vi "Drive_Speed_Set(EEPRM).vi"(1 "Set Speed":i32, 2 "Drive Speed Number":u16(ring) items=["Drive Speed 1", "Drive Speed 2", "Drive Speed 3", "Drive Speed 4"], 3 "Axis":u16(ring) items=["X", "Y"], 4 "baud rate (9600)":u32=115200 caption="보 전송속도(9600)", 5 "Port":refnum<visa-resource-name>="COM4" caption="VISA 리소스 이름") -> (0 "Read Speed":u32)   [LabVIEW 2016]
uses:
  <vilib>/Instr/_visa.llb/VISA Configure Serial Port (Instr).vi
  <vilib>/Instr/_visa.llb/VISA Flush IO Buffer Mask.ctl
panel:
  out "Read Buffer":string
  out "VISA 리소스 이름 출력":refnum<visa-resource-name>
  out "에러 출력":errorcluster
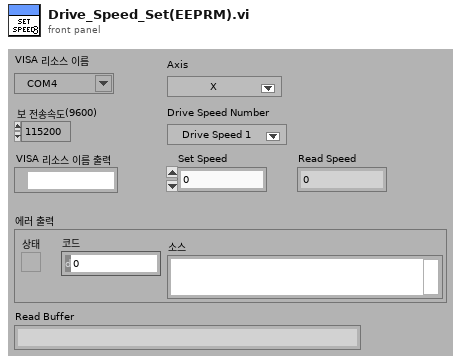
[diagram p1: front panel]
types:
  T1 = typedef "VISA Flush IO Buffer Mask.ctl" = u16
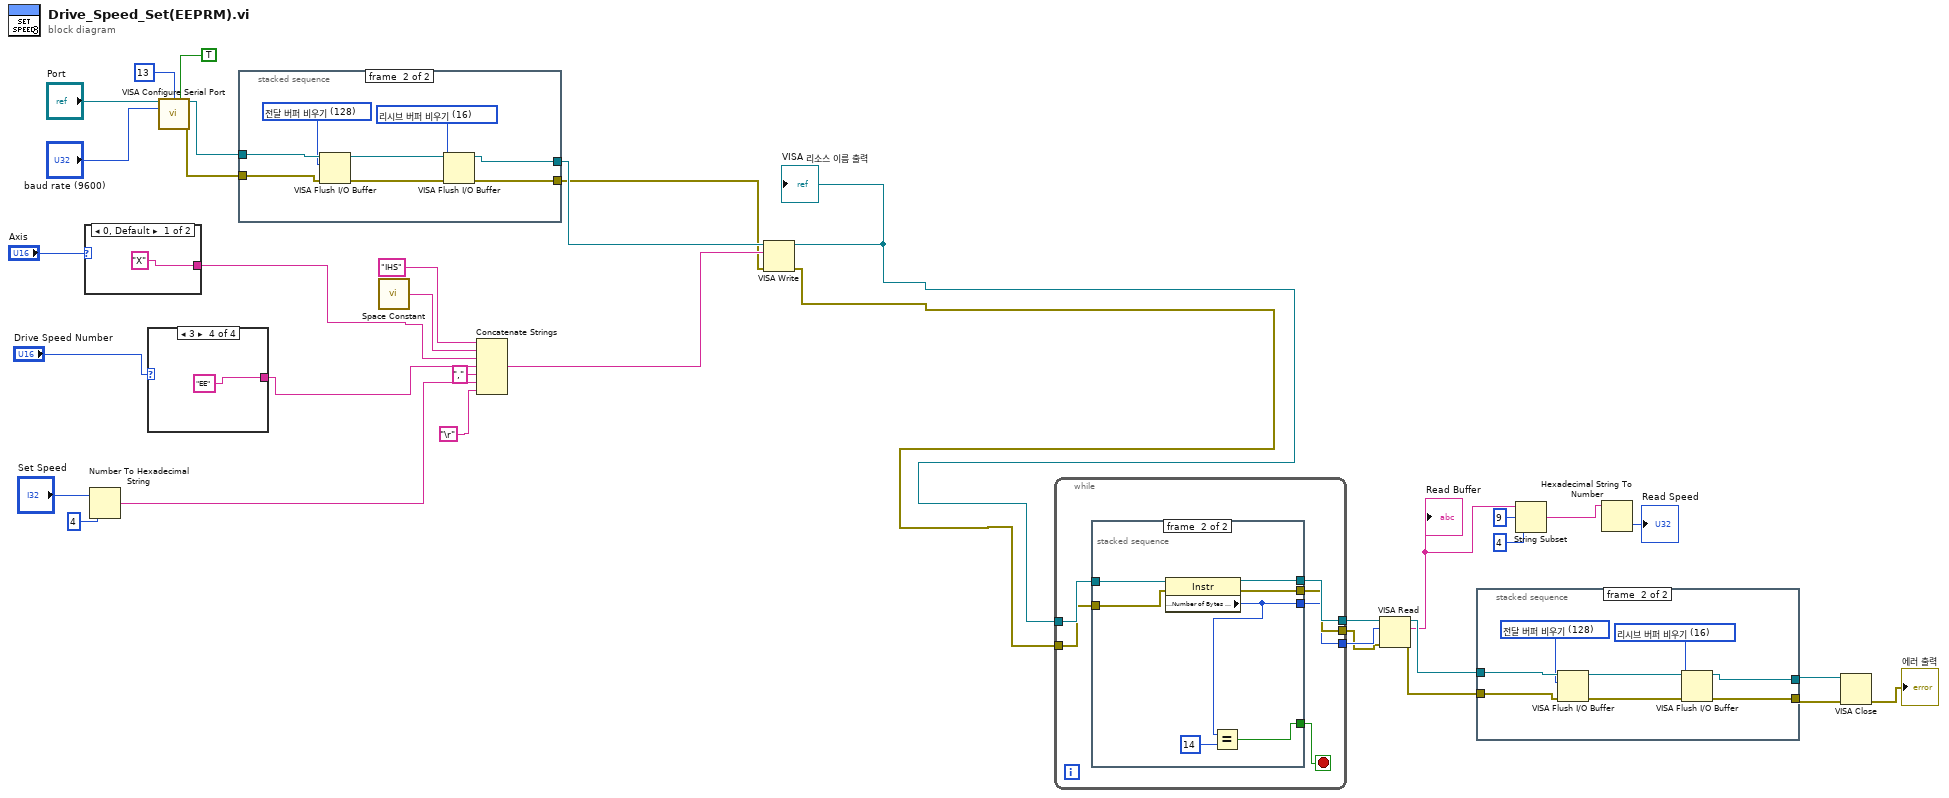
[diagram p0: block diagram]
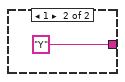
[diagram p2: hidden frame]
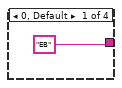
[diagram p3: hidden frame]
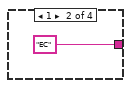
[diagram p4: hidden frame]
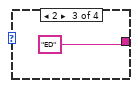
[diagram p5: hidden frame]
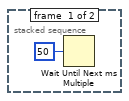
[diagram p6: hidden frame]
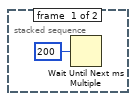
[diagram p7: hidden frame]
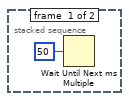
[diagram p8: hidden frame]
diagram:
  n1 = case shown="0, Default" "Axis" {
    tunnel: ["X" ("문자열") "Y" ("문자열")] -> w5
    frame 0, Default {
    }
    frame 1 {
    }
  }
  n2 = Number To Hexadecimal String(1:i16 4 ("폭(-)"), 2:"Set Speed") -> (0:w3:string)
  n3 = case shown="3" "Drive Speed Number" {
    tunnel: ["EB" ("문자열") "EC" ("문자열") "ED" ("문자열") "EE" ("문자열")] -> w13
    frame 0, Default {
    }
    frame 1 {
    }
    frame 2 {
    }
    frame 3 {
    }
  }
  n4 = call-poly "VISA Configure Serial Port"("VISA resource name"="Port", "termination char\n(0xA = '\\n' = LF)"=i16 13 ("termination char\n(0xA = '\\n' = LF)"), "Enable Termination\nChar (T)"=TRUE ("Enable Termination\nChar (T)"), "baud rate (9600)"="baud rate (9600)") -> ("VISA resource name out"=w28:refnum<visa-resource-name>, "error out"=w27:errorcluster)  [unwired: 10 in]
  n5 = stacked-sequence {
    tunnel: w28 -> [_ w50]
    tunnel: w27 -> [_ w49]
    tunnel: [_ w45] -> w26
    tunnel: [_ w44] -> w25
    frame #0 {
      n6 = Wait Until Next ms Multiple(millisecond multiple=u32 50 ("ms 배수")) -> ()  [unwired: 1 out]
    }
    frame #1 {
      w43 = T1 16 items=["리시브 버퍼 비우기"=16, "전달 버퍼 디바이스에 쓰기"=32, "리시브 버퍼 비우기(I/O 없음)"=64, "전달 버퍼 비우기"=128] ("Mask")
      w48 = T1 128 items=["리시브 버퍼 비우기"=16, "전달 버퍼 디바이스에 쓰기"=32, "리시브 버퍼 비우기(I/O 없음)"=64, "전달 버퍼 비우기"=128] ("Mask")
      n7 = VISA Flush I/O Buffer(VISA resource name=w50, mask (16)=w48, error in (no error)=w49) -> (VISA resource name out=w47:refnum<visa-resource-name>, error out=w46:errorcluster)
      n8 = VISA Flush I/O Buffer(VISA resource name=w47, mask (16)=w43, error in (no error)=w46) -> (VISA resource name out=w45:refnum<visa-resource-name>, error out=w44:errorcluster)
    }
  }
  n9 = call <vilib>:"Space Constant.vi"() -> ("String"=w33:string)
  n10 = Concatenate Strings("IHS" ("버퍼 쓰기"), w33, w5, w13, "," ("문자열"), w3, "\r") -> (w34:string)
  n11 = VISA Write(VISA resource name=w26, write buffer=w34, error in (no error)=w25) -> (VISA resource name out=w16:refnum<visa-resource-name>, error out=w15:errorcluster)  [unwired: 1 out]
  "VISA 리소스 이름 출력" <- w16
  n12 = while {
    tunnel: w16 -> [w56]
    tunnel: w15 -> [w55]
    tunnel: [w54] -> w23
    tunnel: [w51] -> w18
    tunnel: [w53] -> w17
    stop <- w52 stop-if-true
    n13 = stacked-sequence {
      tunnel: w56 -> [_ w64]
      tunnel: w55 -> [_ w63]
      tunnel: [_ w62] -> w54
      tunnel: [_ w61] -> w53
      tunnel: [_ w59] -> w52
      tunnel: [_ w58] -> w51
      frame #0 {
        n14 = Wait Until Next ms Multiple(millisecond multiple=u32 200 ("ms 배수")) -> ()  [unwired: 1 out]
      }
      frame #1 {
        n15 = property class="Instr"(reference=w64, error in=w63) -> (reference out=w62:refnum<visa-resource-name>, error out=w61:errorcluster, "Serial Settings:Number of Bytes at Serial Port"=w58:u32)
        n16 = Equal?(x=w58, y=u32 14) -> (x = y?=w59:bool)
      }
    }
  }
  n17 = VISA Read(VISA resource name=w23, byte count=w18, error in (no error)=w17) -> (VISA resource name out=w22:refnum<visa-resource-name>, read buffer=w12:string, error out=w21:errorcluster)  [unwired: 1 out]
  "Read Buffer" <- w12
  n18 = stacked-sequence {
    tunnel: w22 -> [_ w73]
    tunnel: w21 -> [_ w72]
    tunnel: [_ w68] -> w20
    tunnel: [_ w67] -> w19
    frame #0 {
      n19 = Wait Until Next ms Multiple(millisecond multiple=u32 50 ("ms 배수")) -> ()  [unwired: 1 out]
    }
    frame #1 {
      w66 = T1 16 items=["리시브 버퍼 비우기"=16, "전달 버퍼 디바이스에 쓰기"=32, "리시브 버퍼 비우기(I/O 없음)"=64, "전달 버퍼 비우기"=128] ("Mask")
      w71 = T1 128 items=["리시브 버퍼 비우기"=16, "전달 버퍼 디바이스에 쓰기"=32, "리시브 버퍼 비우기(I/O 없음)"=64, "전달 버퍼 비우기"=128] ("Mask")
      n20 = VISA Flush I/O Buffer(VISA resource name=w73, mask (16)=w71, error in (no error)=w72) -> (VISA resource name out=w70:refnum<visa-resource-name>, error out=w69:errorcluster)
      n21 = VISA Flush I/O Buffer(VISA resource name=w70, mask (16)=w66, error in (no error)=w69) -> (VISA resource name out=w68:refnum<visa-resource-name>, error out=w67:errorcluster)
    }
  }
  n22 = String Subset(string=w12, offset (0)=9 ("오프셋(0)"), length (rest)=4 ("길이(나머지)")) -> (substring=w9:string)
  n23 = Hexadecimal String To Number(string=w9) -> (number=→"Read Speed":u32)  [unwired: 2 in, 1 out]
  n24 = VISA Close(VISA resource name=w20, error in (no error)=w19) -> (error out=→"에러 출력":errorcluster)
